vi "acutrol3000.vi"() -> ()   [LabVIEW 2021]
uses:
  event_handler.ctl
  44700b8f-dca4-4afe-b019-5c1f374ad2a9.vi
  b216d5e3-8cc4-4d28-b037-c42745385f66.vi
  fea8172d-1276-46cb-9a99-2a3333d83a4a.vi
  b522c8bc-aa6b-4975-9e05-6c11703ace2c.vi
  16b6a5f6-b29d-406e-b967-7a73e07eb1de.vi
panel:
  in  "Communication":enum16{"TCP", "GPIB"}(ring)
  in  "Save data":bool
  out "String":string="\"Acutronic USA, ACT3000, 1234567890, 01.02.12 (Build 1962)\"\n"
  in  "Query Command":bool
  in  "Send Position":bool
  in  "Send Rate":bool
  in  "Position (deg)":string="0"
  in  "Rate (deg/s)":string="20"
  out "Acceleration":dbl[](graph)=[-0.9243416956465467]
  out "Rate":dbl[](graph)=[0.0001151929704002177]
  out "Position":dbl[](graph)=[72.70071743179678]
  in  "Stop Motion":bool
  in  "Phase":string="0"
  in  "Amplitude (deg)":string="160"
  in  "Frequency (Hz)":string="1"
  in  "Send Oscillation":bool
  in  "Frequency Slew":string="0.01"
  in  "Amplitude Slew":string="2.0"
  in  "file path (dialog if empty)":path
  out "Acquisition period":u32=38
  in  "Send Command":bool
  in  "Command":string="*idn?"
  in  "Stop":bool
  out "Actual State":dbl[](array[numeric])=[72.70071743179678, 0.0001151929704002177, -0.9243416956465467]
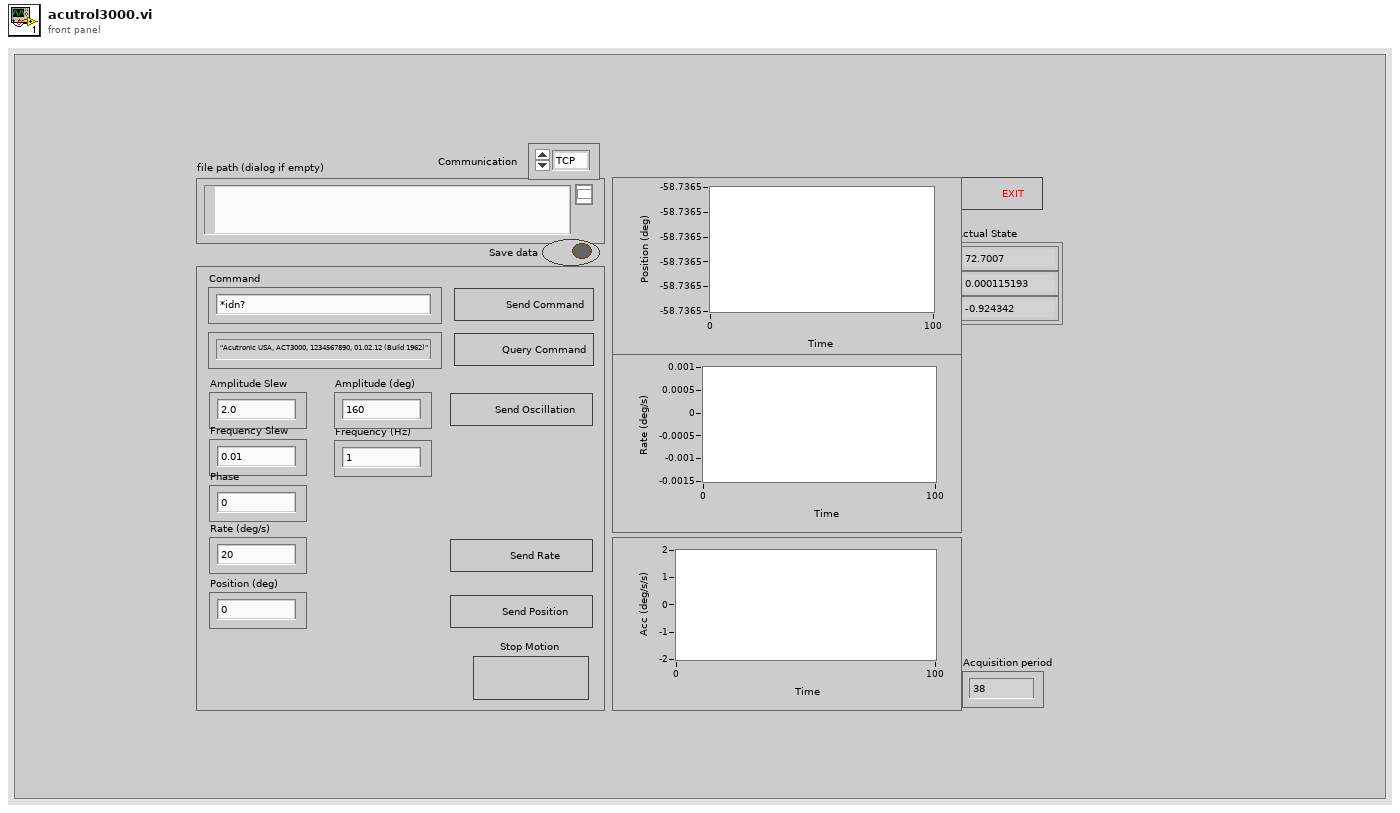
[diagram p1: front panel]
types:
  T1 = typedef "event_handler.ctl" = enum16{"Query Command", "Stop Motion", "Send Oscillation", "Send Position", "Send Rate", "Initialize", "Wait command", "Monitor", "Send command"}
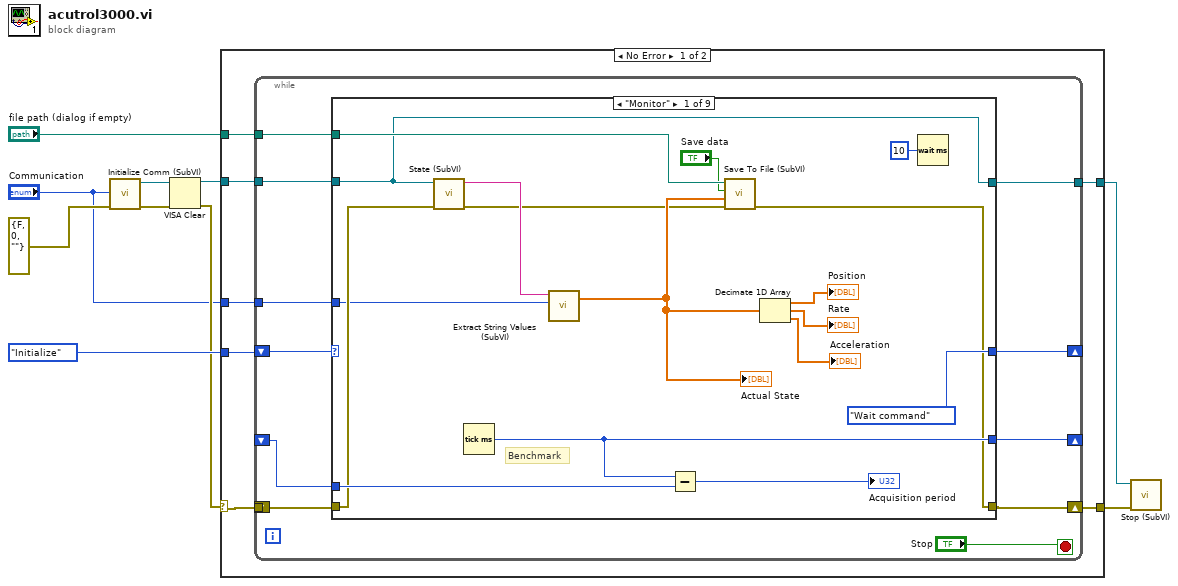
[diagram p0: block diagram]
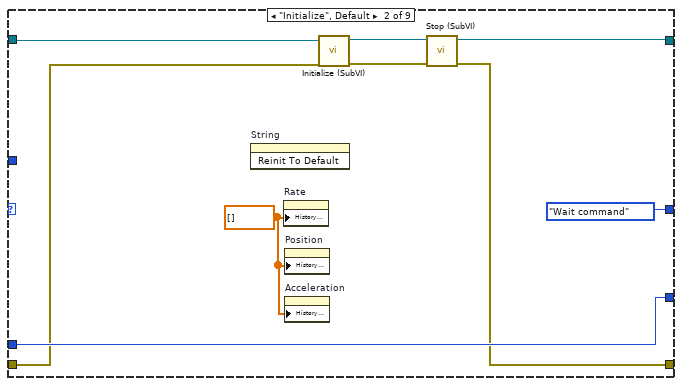
[diagram p2: hidden frame]
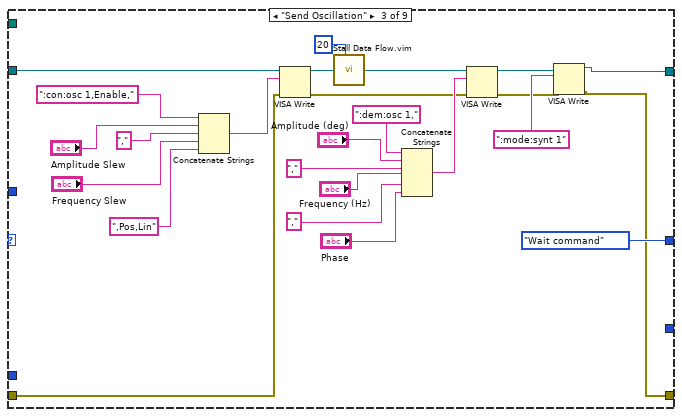
[diagram p3: hidden frame]
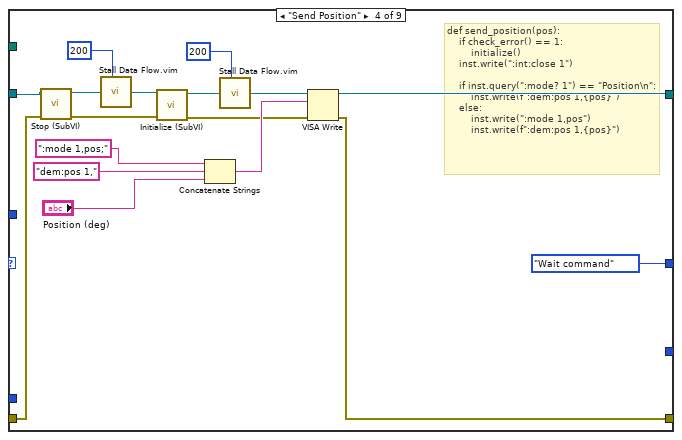
[diagram p4: hidden frame]
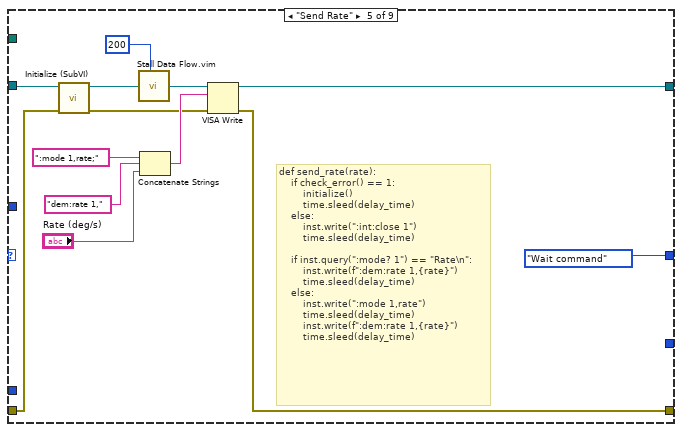
[diagram p5: hidden frame]
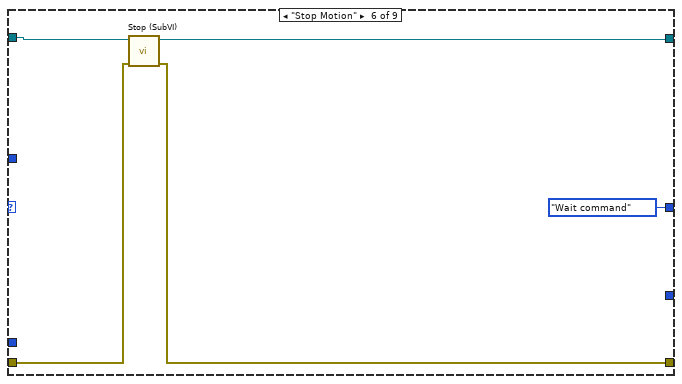
[diagram p6: hidden frame]
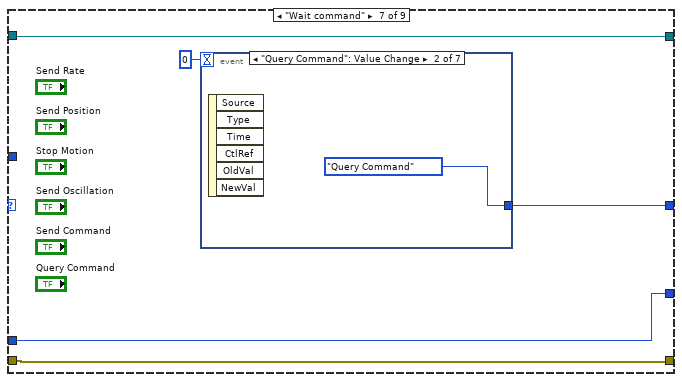
[diagram p7: hidden frame]
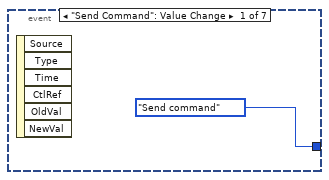
[diagram p8: hidden frame]
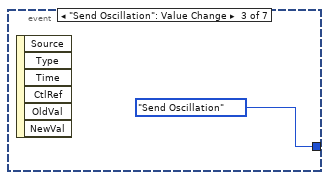
[diagram p9: hidden frame]
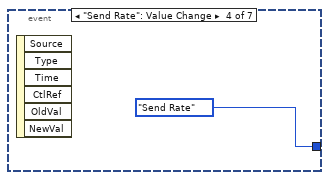
[diagram p10: hidden frame]
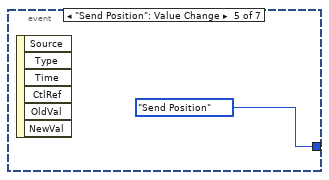
[diagram p11: hidden frame]
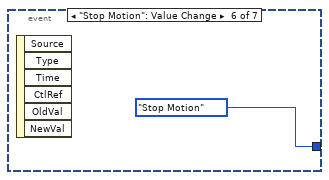
[diagram p12: hidden frame]
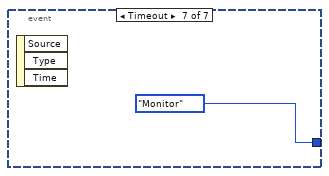
[diagram p13: hidden frame]
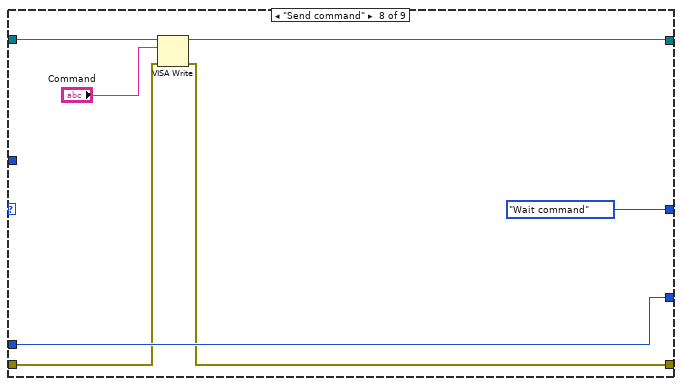
[diagram p14: hidden frame]
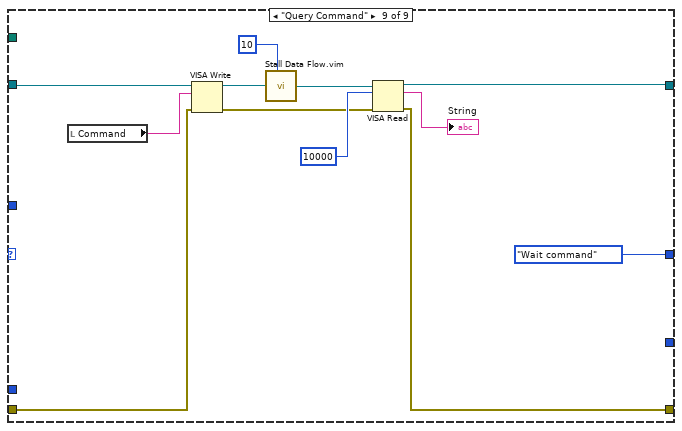
[diagram p15: hidden frame]
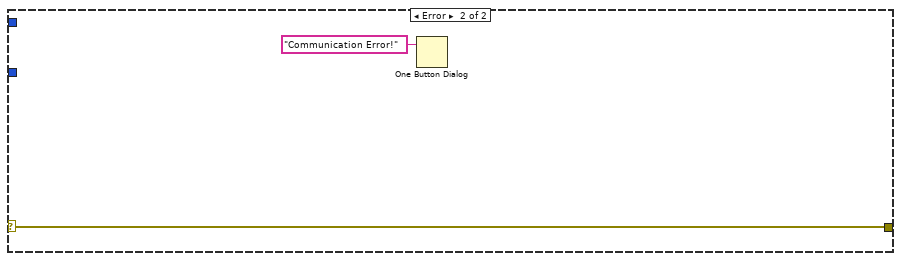
[diagram p16: hidden frame]
diagram:
  n1 = call "Initialize Comm (SubVI).vi"("error in (no error)"=errorcluster {"status"=FALSE, "code"=0, "source"=""}, "Enum"="Communication") -> ("error out"=w3:errorcluster, "reference out"=w2:refnum<visa-resource-name>)  [unwired: 8 in]
  n2 = VISA Clear(VISA resource name=w2, error in (no error)=w3) -> (VISA resource name out=w6:refnum<visa-resource-name>, error out=w5:errorcluster)
  n3 = case shown="No Error" w5 {
    selector: w5 -> [w13 w147]
    tunnel: event_handler."Initialize" -> [w17 _]
    tunnel: "file path (dialog if empty)" -> [w16 _]
    tunnel: w6 -> [w15 _]
    tunnel: [w14 w147] -> w8
    tunnel: [w12 _] -> w7
    tunnel: "Communication" -> [w11 _]
    frame No Error {
      n4 = while {
        tunnel: w15 -> [w26]
        shift-right: [w27] -> _
        shift-left: w17 -> [w28]
        shift-right: [w25] -> _
        shift-left: _ -> [w24]
        tunnel: w16 -> [w23]
        tunnel: w13 -> [w21]
        shift-right: [w22] -> w14
        shift-left: _ -> [_]
        tunnel: [w20] -> w12
        tunnel: w11 -> [w18]
        stop <- "Stop" stop-if-true
        n5 = case shown="\"Monitor\"" w28 {
          tunnel: [event_handler."Wait command" event_handler."Wait command" event_handler."Wait command" event_handler."Wait command" event_handler."Wait command" event_handler."Wait command" w117 event_handler."Wait command" event_handler."Wait command"] -> w27
          tunnel: w26 -> [w32 w47 w79 w89 w108 w114 w115 w131 w138]
          tunnel: [w43 w53 _ _ _ _ w119 w130 _] -> w25
          tunnel: w24 -> [w42 w53 _ _ _ _ w119 w130 _]
          tunnel: w23 -> [w40 _ _ _ _ _ _ _ _]
          tunnel: [w33 w49 w56 w81 w98 w111 w118 w128 w144] -> w22
          tunnel: w21 -> [w35 w46 w59 w84 w100 w112 w118 w129 w135]
          tunnel: [w32 w48 w55 w80 w97 w110 w115 w127 w143] -> w20
          tunnel: w18 -> [w30 _ _ _ _ _ _ _ _]
          frame "Monitor" {
            # "Benchmark"
            n6 = call "State (SubVI).vi"("error in (no error)"=w35, "VISA Refnum in"=w32) -> ("error out"=w34:errorcluster, "read buffer"=w41:string)  [unwired: 8 in]
            n7 = Tick Count (ms)() -> (millisecond timer value=w43:u32)
            n8 = call "Extract String Values (SubVI).vi"("Communication"=w30, "read buffer"=w41) -> ("array type (2D Dbl)"=w39:dbl[])  [unwired: 9 in]
            "Actual State" <- w39
            n9 = Subtract(x=w43, y=w42) -> (x-y=→"Acquisition period":u32)
            n10 = call "Save To File (SubVI).vi"("error in (no error)"=w34, "array type (2D Dbl)"=w39, "Save data"="Save data", "file path (dialog if empty)"=w40) -> ("error out"=w33:errorcluster)  [unwired: 7 in]
            n11 = Decimate 1D Array(w39) -> (→"Position":dbl[], →"Rate":dbl[], →"Acceleration":dbl[])
            n12 = Wait (ms)(milliseconds to wait=u32 10) -> ()  [unwired: 1 out]
          }
          frame "Initialize", Default {
            w51 = dbl[] [] ("History Data")
            n13 = invoke on="String" class="Str" method="Reinit To Default"() -> ()  [unwired: 3 in, 3 out]
            n14 = property on="Rate" class="WFChart (strict)"("History Data"=w51) -> ()  [unwired: 2 in, 2 out]
            n15 = property on="Position" class="WFChart (strict)"("History Data"=w51) -> ()  [unwired: 2 in, 2 out]
            n16 = property on="Acceleration" class="WFChart (strict)"("History Data"=w51) -> ()  [unwired: 2 in, 2 out]
            n17 = call "Initialize (SubVI).vi"("error in (no error)"=w46, "VISA Refnum in"=w47) -> ("error out"=w50:errorcluster, "VISA Refnum out"=w52:refnum<visa-resource-name>)  [unwired: 8 in]
            n18 = call "Stop (SubVI).vi"("error in (no error)"=w50, "VISA Refnum in"=w52) -> ("error out"=w49:errorcluster, "VISA resource name out"=w48:refnum<visa-resource-name>)  [unwired: 8 in]
          }
          frame "Send Oscillation" {
            n19 = Concatenate Strings(":con:osc 1,Enable," ("write buffer"), "Amplitude Slew", "," ("string"), "Frequency Slew", ",Pos,Lin" ("string")) -> (w73:string)
            n20 = VISA Write(VISA resource name=w79, write buffer=w73, error in (no error)=w59) -> (VISA resource name out=w71:refnum<visa-resource-name>, error out=w58:errorcluster)  [unwired: 1 out]
            n21 = call "Stall Data Flow.vim"("value in"=w71, "milliseconds to wait"=u32 20) -> ("value out"=w70:refnum<visa-resource-name>)  [unwired: 1 out]
            n22 = Concatenate Strings(":dem:osc 1," ("write buffer"), "Amplitude (deg)", "," ("string"), "Frequency (Hz)", "," ("string"), "Phase") -> (w62:string)
            n23 = VISA Write(VISA resource name=w70, write buffer=w62, error in (no error)=w58) -> (VISA resource name out=w61:refnum<visa-resource-name>, error out=w57:errorcluster)  [unwired: 1 out]
            n24 = VISA Write(VISA resource name=w61, write buffer=":mode:synt 1", error in (no error)=w57) -> (VISA resource name out=w55:refnum<visa-resource-name>, error out=w56:errorcluster)  [unwired: 1 out]
          }
          frame "Send Position" {
            # "def send_position(pos):\n    if check_error() == 1:\n        initialize()\n    inst.write(\":int:close 1\")\n\n    if inst.query(\":mode? 1\") == \"Position\\n\":\n        inst.write(f\":dem:pos 1,{pos}\")\n    else:\n        inst.write(\":mode 1,pos\")\n        inst.write(f\":dem:pos 1,{pos}\")"
            n25 = call "Stop (SubVI).vi"("error in (no error)"=w84, "VISA Refnum in"=w89) -> ("error out"=w83:errorcluster, "VISA resource name out"=w88:refnum<visa-resource-name>)  [unwired: 8 in]
            n26 = call "Stall Data Flow.vim"("value in"=w88, "milliseconds to wait"=u32 200) -> ("value out"=w87:refnum<visa-resource-name>)  [unwired: 1 out]
            n27 = call "Initialize (SubVI).vi"("error in (no error)"=w83, "VISA Refnum in"=w87) -> ("error out"=w82:errorcluster, "VISA Refnum out"=w95:refnum<visa-resource-name>)  [unwired: 8 in]
            n28 = Concatenate Strings(":mode 1,pos;" ("write buffer"), "dem:pos 1," ("write buffer"), "Position (deg)") -> (w92:string)
            n29 = call "Stall Data Flow.vim"("value in"=w95, "milliseconds to wait"=u32 200) -> ("value out"=w93:refnum<visa-resource-name>)  [unwired: 1 out]
            n30 = VISA Write(VISA resource name=w93, write buffer=w92, error in (no error)=w82) -> (VISA resource name out=w80:refnum<visa-resource-name>, error out=w81:errorcluster)  [unwired: 1 out]
          }
          frame "Send Rate" {
            # "def send_rate(rate):\n    if check_error() == 1:\n        initialize()\n        time.sleed(delay_time)\n    else:\n        inst.write(\":int:close 1\")\n        time.sleed(delay_time)\n\n    if inst.query(\":mode? 1\") == \"Rate\\n\":\n        inst.write(f\":dem:rate 1,{rate}\")\n        time.sleed(delay_time)\n    else:\n        inst.write(\":mode 1,rate\")\n        time.sleed(delay_time)\n        inst.write(f\":dem:rate 1,{rate}\")\n        time.sleed(delay_time)"
            n31 = call "Initialize (SubVI).vi"("error in (no error)"=w100, "VISA Refnum in"=w108) -> ("error out"=w99:errorcluster, "VISA Refnum out"=w107:refnum<visa-resource-name>)  [unwired: 8 in]
            n32 = call "Stall Data Flow.vim"("value in"=w107, "milliseconds to wait"=u32 200) -> ("value out"=w105:refnum<visa-resource-name>)  [unwired: 1 out]
            n33 = Concatenate Strings(":mode 1,rate;" ("write buffer"), "dem:rate 1," ("write buffer"), "Rate (deg/s)") -> (w102:string)
            n34 = VISA Write(VISA resource name=w105, write buffer=w102, error in (no error)=w99) -> (VISA resource name out=w97:refnum<visa-resource-name>, error out=w98:errorcluster)  [unwired: 1 out]
          }
          frame "Stop Motion" {
            n35 = call "Stop (SubVI).vi"("error in (no error)"=w112, "VISA Refnum in"=w114) -> ("error out"=w111:errorcluster, "VISA resource name out"=w110:refnum<visa-resource-name>)  [unwired: 8 in]
          }
          frame "Wait command" {
            n36 = event shown="[1] \"Query Command\": Value Change" {
              selector: _ -> [_ _ _ _ _ _ _]
              dyn-events: _ -> [_ _ _ _ _ _ _]
              timeout: 0 -> [_ _ _ _ _ _ _]
              tunnel: [event_handler."Send command" event_handler."Query Command" event_handler."Send Oscillation" event_handler."Send Rate" event_handler."Send Position" event_handler."Stop Motion" event_handler."Monitor"] -> w117
              event "Send Command": Value Change {
                n37 = event-data() -> ()  [unwired: 1 in, 6 out]
              }
              event "Query Command": Value Change {
                n38 = event-data() -> ()  [unwired: 1 in, 6 out]
              }
              event "Send Oscillation": Value Change {
                n39 = event-data() -> ()  [unwired: 1 in, 6 out]
              }
              event "Send Rate": Value Change {
                n40 = event-data() -> ()  [unwired: 1 in, 6 out]
              }
              event "Send Position": Value Change {
                n41 = event-data() -> ()  [unwired: 1 in, 6 out]
              }
              event "Stop Motion": Value Change {
                n42 = event-data() -> ()  [unwired: 1 in, 6 out]
              }
              event Timeout {
                n43 = event-data() -> ()  [unwired: 1 in, 3 out]
              }
            }
          }
          frame "Send command" {
            n44 = VISA Write(VISA resource name=w131, write buffer="Command", error in (no error)=w129) -> (VISA resource name out=w127:refnum<visa-resource-name>, error out=w128:errorcluster)  [unwired: 1 out]
          }
          frame "Query Command" {
            n45 = local read "Command"() -> (w137:string)
            n46 = VISA Write(VISA resource name=w138, write buffer=w137, error in (no error)=w135) -> (VISA resource name out=w139:refnum<visa-resource-name>, error out=w136:errorcluster)  [unwired: 1 out]
            n47 = call "Stall Data Flow.vim"("value in"=w139, "milliseconds to wait"=u32 10) -> ("value out"=w140:refnum<visa-resource-name>)  [unwired: 1 out]
            n48 = VISA Read(VISA resource name=w140, byte count=u32 10000, error in (no error)=w136) -> (VISA resource name out=w143:refnum<visa-resource-name>, read buffer=→"String":string, error out=w144:errorcluster)  [unwired: 1 out]
          }
        }
      }
    }
    frame Error {
      n49 = One Button Dialog(message="Communication Error!") -> ()  [unwired: 1 in, 1 out]
    }
  }
  n50 = call "Stop (SubVI).vi"("error in (no error)"=w8, "VISA Refnum in"=w7) -> ()  [unwired: 8 in, 2 out]
